vi "example_move_motor_to_position.vi"() -> ()   [LabVIEW 2012]
doc: "EXAMPLE: Move To Target\n\nThis example VI moves the motor to a desired target position. If that position should exceed the counter limitations of the motor, an error will be triggered and the move will not take place.\n\nFurthermore, the VI issues an enable command before attempting the move (to be sure the motor is actually ready to move).\n\nProduced By:\n\nChristopher Lemieux\nKod Integrations, LLC\n4835 Marianne Drive\nMount Airy, MD 21771\nhttp://www.kodintegrations.com\nemail: clemieux@kodintegrations.com\nphone: (240) 687-1288"
uses:
  main_functions/commands.ctl
panel:
  out "current_position (prior to move)":i32
  in  "New Position:":i32
  in  "device_index (def=0)":i32
  out "error out":errorcluster
  in  "error in (no error)":errorcluster
  # "To Operate:\n\n(1) Enter the Device Index. If only one is connected\nthen leave as the default (0)\n\n(2) Enter the new position to move the motor to.  Be sure\nit's not the same position where the motor currently sits\n\n(3) click the arrow button to run the VI\n\n(4) allow movement to complete before stopping VI, otherwise\nthe connection will not be properly terminated"
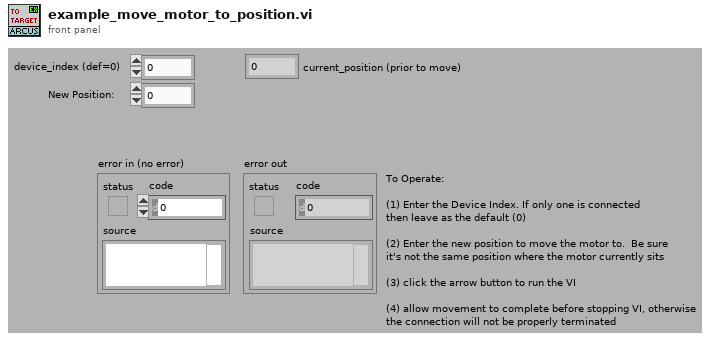
[diagram p1: front panel]
types:
  T1 = typedef "commands.ctl" = enum16{"clearErr", "constJogNeg", "constJogPos", "getAccel", "getActualAmp", "getDeviceId", "getDigInputStatus", "getDigInputsStatus", "getDigOutputStatus", "getDigOutputsStatus", "getFirmwareVer", "getHighSpeed", "getIdleAmp", "getLowSpeed", "getMicroStep", "getMotorStatus", "getMoveMode", "getPolarity", "getPosition", "getProdId", "getPwrStatus", "getRunAmp", "getStatus", "homeNeg", "homePos", "moveToPosition", "powerDown", "powerUp", "setAccel", "setDeviceId", "setDigOutput", "setDigOutputs", "setHighSpeed", "setIdleAmp", "setLowSpeed", "setMoveModeAbs", "setMoveModeIncr", "setPolarity", "setPosition", "setRunAmp", "stopNow", "stopSlow", "storeToMem"}
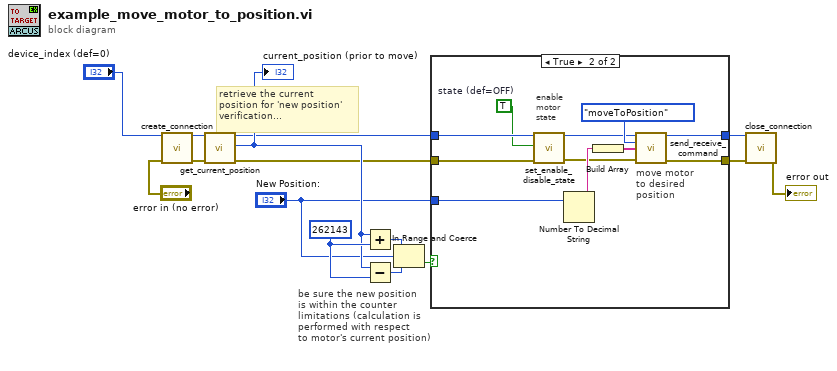
[diagram p0: block diagram]
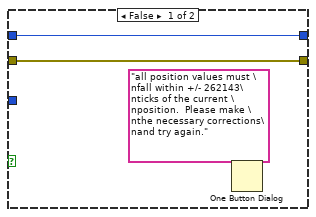
[diagram p2: hidden frame]
diagram:
  w8 = 262143
  # "retrieve the current\nposition for 'new position'\nverification..."
  # "be sure the new position\nis within the counter \nlimitations (calculation is\nperformed with respect\nto motor's current position)"
  n1 = call "create_connection.vi"("device_index (def=0)"="device_index (def=0)", "error in (no error)"="error in (no error)") -> ("reference"=w12:i32, "error out"=w11:errorcluster)  [unwired: 12 in]
  n2 = call "get_current_position.vi"("reference (in)"=w12, "error in (no error)"=w11) -> ("reference (dup)"=w4:i32, "current_position (units)"=w7:i32, "error out"=w6:errorcluster)  [unwired: 15 in]
  "current_position (prior to move)" <- w7
  n3 = Add(x=w7, y=w8) -> (x+y=w10:i32)
  n4 = Subtract(x=w7, y=w8) -> (x-y=w9:i32)
  n5 = In Range and Coerce(upper limit=w10, x="New Position:", lower limit=w9) -> (In Range?=w5:bool)  [unwired: 1 out]
  n6 = case shown="True" w5 {
    tunnel: w6 -> [w18 w24]
    tunnel: [w18 w19] -> w1
    tunnel: w4 -> [w16 w25]
    tunnel: [w16 w20] -> w2
    tunnel: "New Position:" -> [_ w28]
    frame False {
      n7 = One Button Dialog(message="all position values must \nfall within +/- 262143\nticks of the current \nposition.  Please make \nthe necessary corrections\nand try again.") -> ()  [unwired: 1 in, 1 out]
    }
    frame True {
      w23 = TRUE  # state (def=OFF)
      # "move motor\nto desired\nposition"
      # "enable\nmotor\nstate"
      n8 = call "set_enable_disable_state.vi"("reference (in)"=w25, "state (def=OFF)"=w23, "error in (no error)"=w24) -> ("reference (dup)"=w21:i32, "error out"=w22:errorcluster)  [unwired: 14 in, 1 out]
      n9 = Number To Decimal String(number=w28) -> (decimal integer string=w27:string)  [unwired: 1 in]
      n10 = Build Array(w27) -> (w26:string[])
      n11 = call "send_receive_command.vi"("reference (in)"=w21, "command"=commands."moveToPosition", "params (opt)"=w26, "error in (no error)"=w22) -> ("reference (dup)"=w20:i32, "error out"=w19:errorcluster)  [unwired: 7 in, 3 out]
    }
  }
  n12 = call "close_connection.vi"("reference"=w2, "error in (no error)"=w1) -> ("error out"=→"error out":errorcluster)  [unwired: 13 in]
